vi "get device name.vi"(8 "error in (no error)":errorcluster, 11 "DeviceIndex":u32) -> (0 "error out":errorcluster, 3 "Device Name":string)   [LabVIEW 2015, in "rtlsdr.lvlib"]
doc: "Gets the name of the device specified by <index>"
uses:
  rtlsdr.lvlib
  rtlsdr/rtlsdr.dll
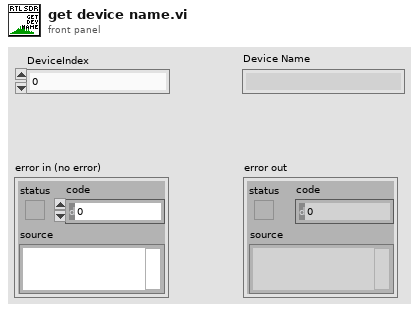
[diagram p1: front panel]
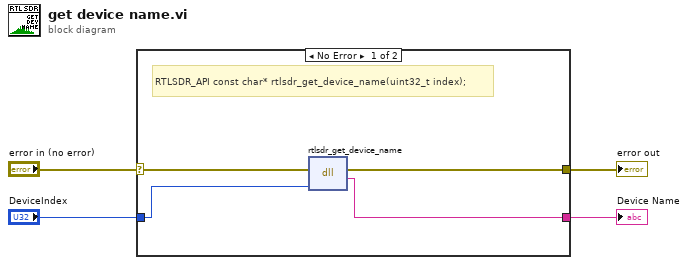
[diagram p0: block diagram]
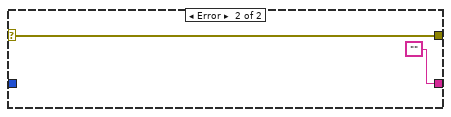
[diagram p2: hidden frame]
diagram:
  n1 = case shown="No Error" "error in (no error)" {
    selector: "error in (no error)" -> [w5 w9]
    tunnel: [w8 ""] -> w4
    tunnel: "DeviceIndex" -> [w7 _]
    tunnel: [w6 w9] -> w1
    frame No Error {
      # "RTLSDR_API const char* rtlsdr_get_device_name(uint32_t index);"
      n2 = dll-call lib="C:/Users/TheDoctor/Documents/Projects/Labview Libraries/rtlsdr/rtlsdr.*" fn="rtlsdr_get_device_name"(error in=w5, "index"=w7) -> (error out=w6:errorcluster, "return type"=w8:string)  [unwired: 3 in, 1 out]
    }
    frame Error {
    }
  }
  "Device Name" <- w4
  "error out" <- w1
